vi "Shutdown.vi"(8 "error in":errorcluster, 11 "Modbus master in":refnum<class "Modbus Master.lvclass">) -> (0 "error out":errorcluster)   [LabVIEW 2013, in "Modbus Library - Advance.lvlib" / "Modbus Master.lvclass"]
doc: "Performs any actions needed to shutdown and clean up the Modbus instance provided. For a Modbus master, this requires closing the connection to the physical bus."
uses:
  Modbus Master.lvclass
  Modbus Master.lvclass/Modbus Master.ctl
  Network Protocol/Network Master/Network Master.lvclass
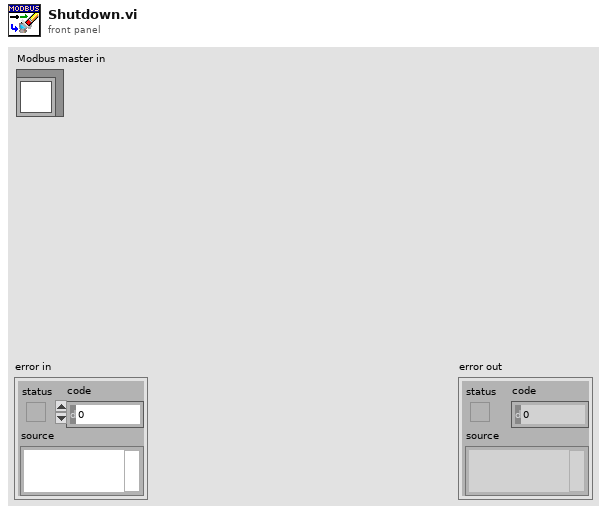
[diagram p1: front panel]
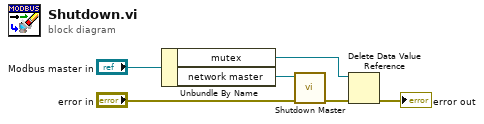
[diagram p0: block diagram]
diagram:
  n1 = Unbundle By Name("Modbus master in") -> ("mutex"=w3:refnum<data-value>, "network master"=w5:refnum<class "Network Master.lvclass">)
  n2 = call-dynamic "Shutdown Master.vi"("error in"="error in", "Network Master in"=w5) -> ("error out"=w2:errorcluster)  [unwired: 8 in, 1 out]
  n3 = Delete Data Value Reference(data value reference=w3, error in=w2) -> (error out=→"error out":errorcluster)  [unwired: 1 out]
